vi "InitializeFile.vi"(0 "File Path":path=path "C:/Users/lbignell/Desktop/1 Ton Tank Experiment/Control Software/HDF5/Dummy2.h5", 1 "Thermocouple Location":string[](array[string])=["In Dark Box", "In Room"], 2 "Multiplicity Requirement":u8 max=8, 3 "Run Number":i32, 4 "VME Configuration":T1={"Module Description"=["Bridge", "TDC", "Scaler", "Hodoscope QDC ", "Other QDC", "Digitizer 1", "Digitizer 2", ""], "Module Model"=["V2718", "V775", "V830", "V965A", "V965A", "V1729A", "1729A", ""], "Module Address"=[0, 4026597376, 4026662912, 4026728448, 4026793984, 4026859520, 4026925056]} {"Module Address" format="%.0x"}, 5 "Trigger Bit Descriptions":string[](array[string])=["TrigA", "TrigB", "TrigC", "TrigD"], 6 "LED Frequency (Hz)":dbl, 7 "error in":errorcluster, 8 "Scaler Info":T3={"Chanel Description"=["H0", "H1", "H2", "H3", "H4", "H5", "TrigA", "TrigB", "TrigC", "TrigD", "Ch0", "Ch1", "Ch2", "Ch3", "Ch4", "Ch5", "Ch6", "Ch7"], "Only Hodo?"=[TRUE, TRUE, TRUE, TRUE, TRUE, TRUE, TRUE, TRUE, FALSE, FALSE, FALSE, FALSE, FALSE, FALSE, FALSE, FALSE, FALSE, FALSE]}, 9 "Optional Comments":string, 12 "HV Status":bool, 13 "Material in Tank":string(combo), 14 "Run Type":string(combo), 15 "TDC Info":T3={"Chanel Description"=["H0", "H1", "H2", "H3", "H4", "H5", "TrigA", "TrigB", "TrigC", "TrigD"], "Only Hodo?"=[TRUE, TRUE, TRUE, TRUE, TRUE, TRUE, TRUE, TRUE, FALSE, FALSE]}, 16 "QDC Info":T3={"Chanel Description"=["H0", "H1", "H2", "H3", "H4", "H5"], "Only Hodo?"=[TRUE, TRUE, TRUE, TRUE, TRUE, TRUE]}, 17 "Digitizer Info":T3={"Chanel Description"=["Ch0", "Ch1", "Ch2", "Ch3", "Ch4", "Ch5", "Ch6", "Ch7"], "Only Hodo?"=[FALSE, FALSE, FALSE, FALSE, FALSE, FALSE, FALSE, FALSE]}) -> (20 "File Handle":T2=16777216 format="%.0x", 27 "error out":errorcluster)   [LabVIEW 2014]
uses:
  <vilib>/addons/h5labview2/base/hid_t.ctl
  <vilib>/addons/h5labview2/file/H5Fmode.ctl
  <vilib>/addons/h5labview2/base/lib_path.vi
  <vilib>/addons/h5labview2/base/H5Equery.vi
  DatasetNames.vi
  <vilib>/addons/h5labview2/dataset/H5Dwrite.llb/H5Dwrite.xnode
  <vilib>/addons/h5labview2/file/H5F.lvlib
  <vilib>/addons/h5labview2/group/H5G.lvlib
  <vilib>/addons/h5labview2/props/H5P.lvlib
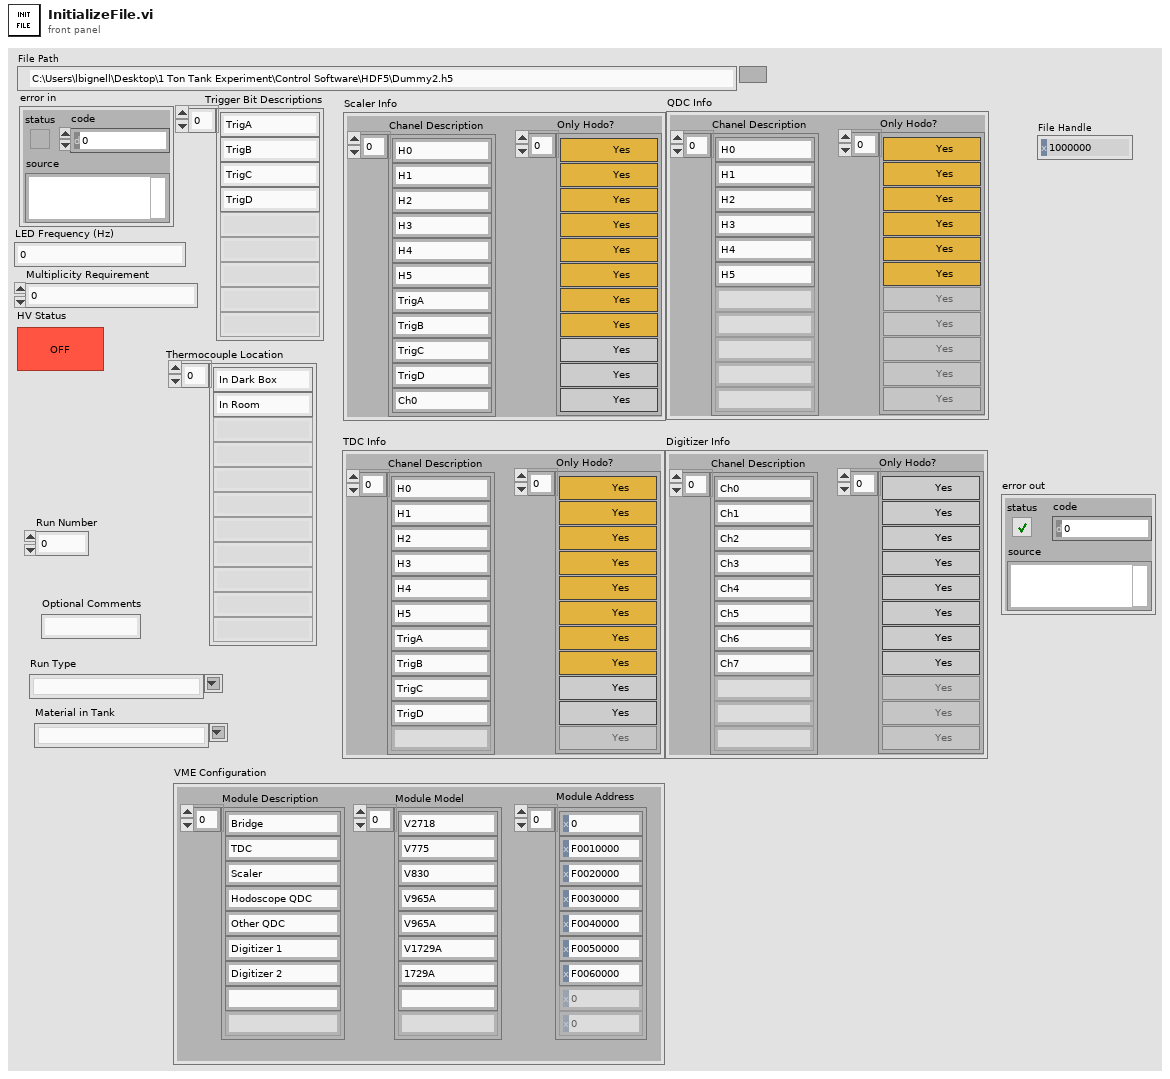
[diagram p1: front panel]
types:
  T1 = cluster{"Module Description":string[], "Module Model":string[], "Module Address":u32[]}
  T2 = typedef "hid_t.ctl" = i32
  T3 = cluster{"Chanel Description":string[], "Only Hodo?":bool[]}
  T4 = typedef "H5F.lvlib/H5Fmode.ctl" = enum16{"read-only", "read-write", "overwrite", "create new", "open or create"}
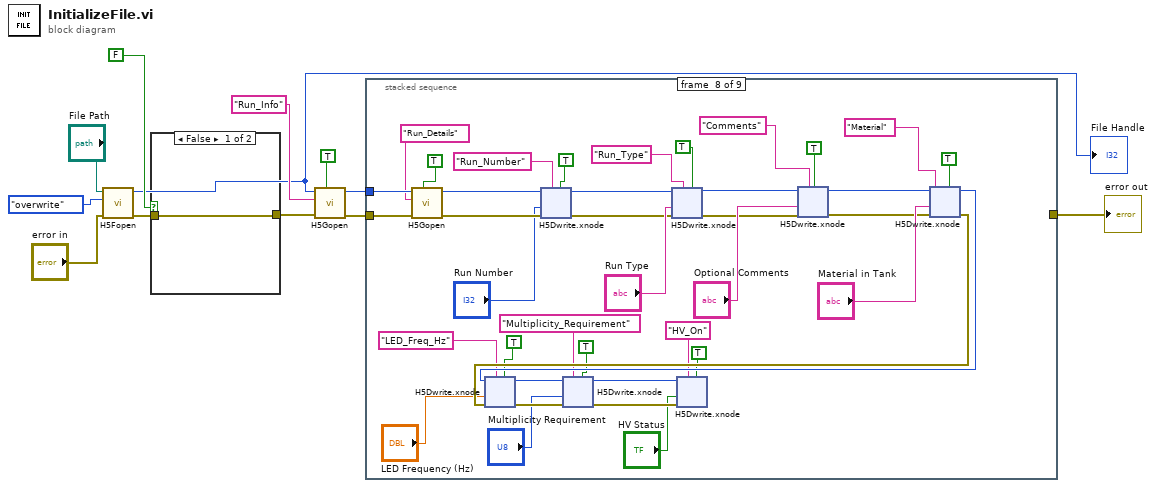
[diagram p0: block diagram]
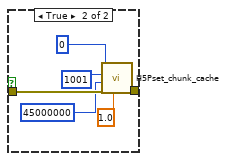
[diagram p2: hidden frame]
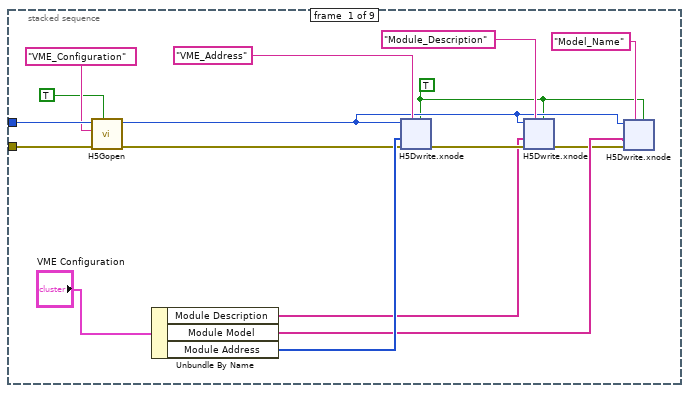
[diagram p3: hidden frame]
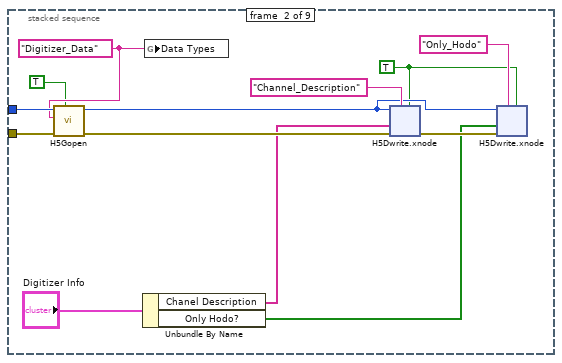
[diagram p4: hidden frame]
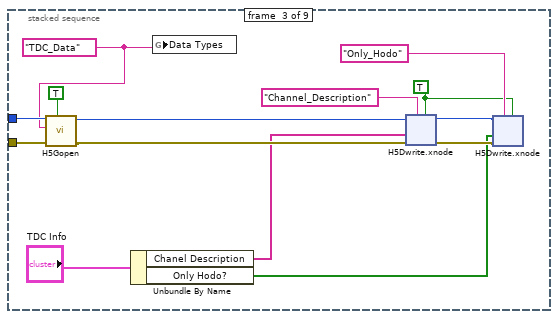
[diagram p5: hidden frame]
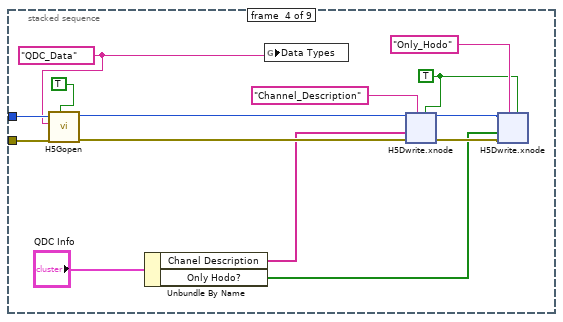
[diagram p6: hidden frame]
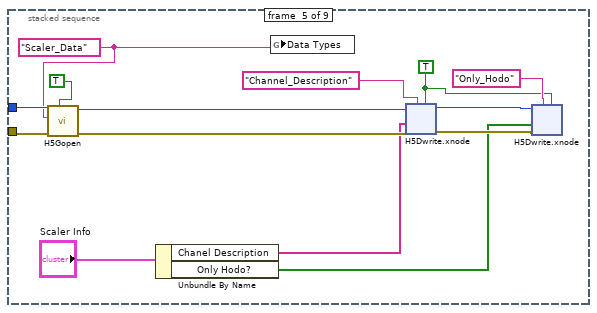
[diagram p7: hidden frame]
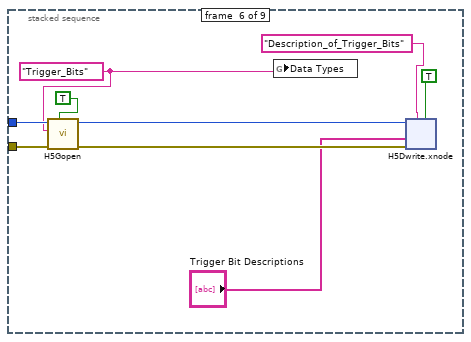
[diagram p8: hidden frame]
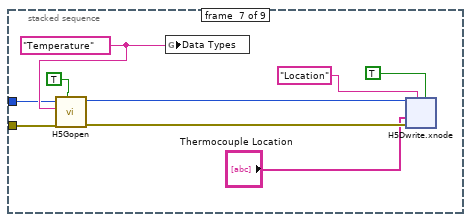
[diagram p9: hidden frame]
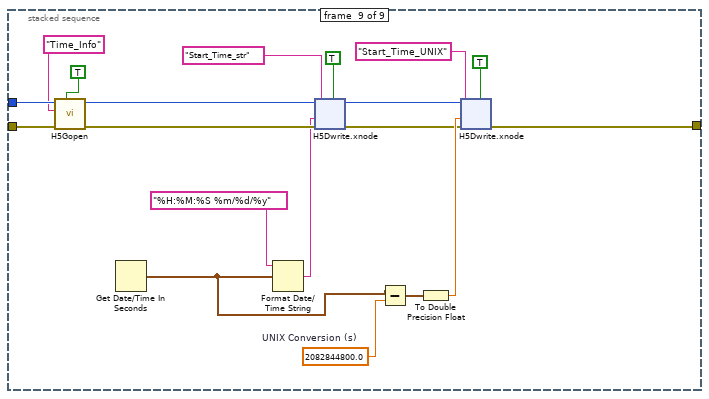
[diagram p10: hidden frame]
diagram:
  n1 = call <vilib>:"H5Fopen.vi"("error in (no error)"="error in", "mode (read-only)"=H5Fmode."overwrite", "path"="File Path") -> ("error out"=w4:errorcluster, "ref out"=w1:T2)  [unwired: 7 in]
  "File Handle" <- w1
  n2 = case shown="False" FALSE {
    tunnel: w4 -> [w13 w19]
    tunnel: [w13 w18] -> w3
    frame False {
    }
    frame True {
      n3 = call <vilib>:"H5Pset_chunk_cache.vi"("w0"=1.0, "error in (no error)"=w19, "nbytes"=u32 45000000, "nslots"=u32 1001, "prop in"=T2 0) -> ("error out"=w18:errorcluster)  [unwired: 5 in, 1 out]
    }
  }
  n4 = call <vilib>:"H5Gopen.vi"("create? (F)"=TRUE, "error in (no error)"=w3, "name"="Run_Info", "ref in"=w1) -> ("error out"=w7:errorcluster, "group out"=w8:T2)  [unwired: 6 in]
  n5 = stacked-sequence {
    tunnel: w8 -> [w31 w100 w149 w200 w250 w296 w317 w380 w525]
    tunnel: w7 -> [w32 w101 w151 w201 w251 w295 w323 w381 w526]
    tunnel: [_ _ _ _ _ _ _ _ w508] -> w6
    frame #0 {
      w21 = TRUE ("replace? (F)")
      n6 = call <vilib>:"H5Gopen.vi"("create? (F)"=TRUE, "error in (no error)"=w32, "name"="VME_Configuration" ("attrib name"), "ref in"=w31) -> ("error out"=w29:errorcluster, "group out"=w25:T2)  [unwired: 6 in]
      n7 = Unbundle By Name("VME Configuration") -> ("Module Description"=w26:string[], "Module Model"=w23:string[], "Module Address"=w33:u32[])
      n8 = xnode "H5Dwrite.xnode"("replace? (F)"=w21, "dataset name"="VME_Address" ("attrib name"), "error in (no error)"=w29, "data"=w33, "ref in"=w25) -> ("error out"=w27:errorcluster)  [unwired: 2 in, 2 out]
      n9 = xnode "H5Dwrite.xnode"("replace? (F)"=w21, "dataset name"="Module_Description" ("attrib name"), "error in (no error)"=w27, "data"=w26, "ref in"=w25) -> ("error out"=w22:errorcluster)  [unwired: 2 in, 2 out]
      n10 = xnode "H5Dwrite.xnode"("replace? (F)"=w21, "dataset name"="Model_Name" ("attrib name"), "error in (no error)"=w22, "data"=w23, "ref in"=w25) -> ()  [unwired: 2 in, 3 out]
    }
    frame #1 {
      w98 = "Digitizer_Data" ("Combo Box")
      w92 = TRUE ("replace? (F)")
      n11 = call <vilib>:"H5Gopen.vi"("create? (F)"=TRUE, "error in (no error)"=w101, "name"=w98, "ref in"=w100) -> ("error out"=w99:errorcluster, "group out"=w94:T2)  [unwired: 6 in]
      n12 = Unbundle By Name("Digitizer Info") -> ("Chanel Description"=w96:string[], "Only Hodo?"=w91:bool[])
      n13 = global write "DatasetNames.vi" "Data Types"(w98) -> ()
      n14 = xnode "H5Dwrite.xnode"("replace? (F)"=w92, "dataset name"="Channel_Description" ("attrib name"), "error in (no error)"=w99, "data"=w96, "ref in"=w94) -> ("error out"=w95:errorcluster)  [unwired: 2 in, 2 out]
      n15 = xnode "H5Dwrite.xnode"("replace? (F)"=w92, "dataset name"="Only_Hodo" ("attrib name"), "error in (no error)"=w95, "data"=w91, "ref in"=w94) -> ()  [unwired: 2 in, 3 out]
    }
    frame #2 {
      w140 = TRUE ("replace? (F)")
      w148 = "TDC_Data" ("Combo Box")
      n16 = call <vilib>:"H5Gopen.vi"("create? (F)"=TRUE, "error in (no error)"=w151, "name"=w148, "ref in"=w149) -> ("error out"=w150:errorcluster, "group out"=w145:T2)  [unwired: 6 in]
      n17 = Unbundle By Name("TDC Info") -> ("Chanel Description"=w144:string[], "Only Hodo?"=w139:bool[])
      n18 = global write "DatasetNames.vi" "Data Types"(w148) -> ()
      n19 = xnode "H5Dwrite.xnode"("replace? (F)"=w140, "dataset name"="Channel_Description" ("attrib name"), "error in (no error)"=w150, "data"=w144, "ref in"=w145) -> ("error out"=w143:errorcluster, "ref out"=w142:i32)  [unwired: 2 in, 1 out]
      n20 = xnode "H5Dwrite.xnode"("replace? (F)"=w140, "dataset name"="Only_Hodo" ("attrib name"), "error in (no error)"=w143, "data"=w139, "ref in"=w142) -> ()  [unwired: 2 in, 3 out]
    }
    frame #3 {
      w190 = TRUE ("replace? (F)")
      w197 = "QDC_Data" ("Combo Box")
      n21 = call <vilib>:"H5Gopen.vi"("create? (F)"=TRUE ("replace? (F)"), "error in (no error)"=w201, "name"=w197, "ref in"=w200) -> ("error out"=w198:errorcluster, "group out"=w199:T2)  [unwired: 6 in]
      n22 = Unbundle By Name("QDC Info") -> ("Chanel Description"=w194:string[], "Only Hodo?"=w189:bool[])
      n23 = global write "DatasetNames.vi" "Data Types"(w197) -> ()
      n24 = xnode "H5Dwrite.xnode"("replace? (F)"=w190, "dataset name"="Channel_Description" ("attrib name"), "error in (no error)"=w198, "data"=w194, "ref in"=w199) -> ("error out"=w193:errorcluster, "ref out"=w192:i32)  [unwired: 2 in, 1 out]
      n25 = xnode "H5Dwrite.xnode"("replace? (F)"=w190, "dataset name"="Only_Hodo" ("attrib name"), "error in (no error)"=w193, "data"=w189, "ref in"=w192) -> ()  [unwired: 2 in, 3 out]
    }
    frame #4 {
      w239 = TRUE ("replace? (F)")
      w247 = "Scaler_Data" ("Combo Box")
      n26 = call <vilib>:"H5Gopen.vi"("create? (F)"=TRUE, "error in (no error)"=w251, "name"=w247, "ref in"=w250) -> ("error out"=w248:errorcluster, "group out"=w249:T2)  [unwired: 6 in]
      n27 = Unbundle By Name("Scaler Info") -> ("Chanel Description"=w244:string[], "Only Hodo?"=w240:bool[])
      n28 = global write "DatasetNames.vi" "Data Types"(w247) -> ()
      n29 = xnode "H5Dwrite.xnode"("replace? (F)"=w239, "dataset name"="Channel_Description" ("attrib name"), "error in (no error)"=w248, "data"=w244, "ref in"=w249) -> ("error out"=w243:errorcluster, "ref out"=w242:i32)  [unwired: 2 in, 1 out]
      n30 = xnode "H5Dwrite.xnode"("replace? (F)"=w239, "dataset name"="Only_Hodo" ("attrib name"), "error in (no error)"=w243, "data"=w240, "ref in"=w242) -> ()  [unwired: 2 in, 3 out]
    }
    frame #5 {
      w292 = "Trigger_Bits" ("Combo Box")
      n31 = call <vilib>:"H5Gopen.vi"("create? (F)"=TRUE ("replace? (F)"), "error in (no error)"=w295, "name"=w292, "ref in"=w296) -> ("error out"=w294:errorcluster, "group out"=w293:T2)  [unwired: 6 in]
      n32 = global write "DatasetNames.vi" "Data Types"(w292) -> ()
      n33 = xnode "H5Dwrite.xnode"("replace? (F)"=TRUE, "dataset name"="Description_of_Trigger_Bits" ("attrib name"), "error in (no error)"=w294, "data"="Trigger Bit Descriptions", "ref in"=w293) -> ()  [unwired: 2 in, 3 out]
    }
    frame #6 {
      w321 = "Temperature" ("Combo Box")
      n34 = call <vilib>:"H5Gopen.vi"("create? (F)"=TRUE ("replace? (F)"), "error in (no error)"=w323, "name"=w321, "ref in"=w317) -> ("error out"=w322:errorcluster, "group out"=w316:T2)  [unwired: 6 in]
      n35 = global write "DatasetNames.vi" "Data Types"(w321) -> ()
      n36 = xnode "H5Dwrite.xnode"("replace? (F)"=TRUE, "dataset name"="Location" ("attrib name"), "error in (no error)"=w322, "data"="Thermocouple Location", "ref in"=w316) -> ()  [unwired: 2 in, 3 out]
    }
    frame #7 {
      n37 = call <vilib>:"H5Gopen.vi"("create? (F)"=TRUE, "error in (no error)"=w381, "name"="Run_Details", "ref in"=w380) -> ("error out"=w361:errorcluster, "group out"=w363:T2)  [unwired: 6 in]
      n38 = xnode "H5Dwrite.xnode"("replace? (F)"=TRUE, "dataset name"="Run_Number", "error in (no error)"=w361, "data"="Run Number", "ref in"=w363) -> ("error out"=w362:errorcluster, "ref out"=w364:i32)  [unwired: 2 in, 1 out]
      n39 = xnode "H5Dwrite.xnode"("replace? (F)"=TRUE, "dataset name"="Run_Type", "error in (no error)"=w362, "data"="Run Type", "ref in"=w364) -> ("error out"=w373:errorcluster, "ref out"=w372:i32)  [unwired: 2 in, 1 out]
      n40 = xnode "H5Dwrite.xnode"("replace? (F)"=TRUE, "dataset name"="Comments", "error in (no error)"=w373, "data"="Optional Comments", "ref in"=w372) -> ("error out"=w368:errorcluster, "ref out"=w369:i32)  [unwired: 2 in, 1 out]
      n41 = xnode "H5Dwrite.xnode"("replace? (F)"=TRUE, "dataset name"="Material", "error in (no error)"=w368, "data"="Material in Tank", "ref in"=w369) -> ("error out"=w356:errorcluster, "ref out"=w357:i32)  [unwired: 2 in, 1 out]
      n42 = xnode "H5Dwrite.xnode"("replace? (F)"=TRUE, "dataset name"="LED_Freq_Hz", "error in (no error)"=w356, "data"="LED Frequency (Hz)", "ref in"=w357) -> ("error out"=w351:errorcluster, "ref out"=w350:i32)  [unwired: 2 in, 1 out]
      n43 = xnode "H5Dwrite.xnode"("replace? (F)"=TRUE, "dataset name"="Multiplicity_Requirement", "error in (no error)"=w351, "data"="Multiplicity Requirement", "ref in"=w350) -> ("error out"=w347:errorcluster, "ref out"=w346:i32)  [unwired: 2 in, 1 out]
      n44 = xnode "H5Dwrite.xnode"("replace? (F)"=TRUE, "dataset name"="HV_On", "error in (no error)"=w347, "data"="HV Status", "ref in"=w346) -> ()  [unwired: 2 in, 3 out]
    }
    frame #8 {
      w517 = 2082844800.0  # UNIX Conversion (s)
      n45 = call <vilib>:"H5Gopen.vi"("create? (F)"=TRUE, "error in (no error)"=w526, "name"="Time_Info", "ref in"=w525) -> ("error out"=w521:errorcluster, "group out"=w522:T2)  [unwired: 6 in]
      n46 = Get Date/Time In Seconds() -> (seconds since 1Jan1904=w516:timestamp)
      n47 = Format Date/Time String(time format string (%c)="%H:%M:%S %m/%d/%y", seconds (now)=w516) -> (date/time string=w518:string)  [unwired: 1 in]
      n48 = xnode "H5Dwrite.xnode"("replace? (F)"=TRUE, "dataset name"="Start_Time_str", "error in (no error)"=w521, "data"=w518, "ref in"=w522) -> ("error out"=w512:errorcluster, "ref out"=w513:i32)  [unwired: 2 in, 1 out]
      n49 = Subtract(x=w516, y=w517) -> (x-y=w515:timestamp)
      n50 = To Double Precision Float(number=w515) -> (double precision float=w514:dbl)
      n51 = xnode "H5Dwrite.xnode"("replace? (F)"=TRUE, "dataset name"="Start_Time_UNIX", "error in (no error)"=w512, "data"=w514, "ref in"=w513) -> ("error out"=w508:errorcluster)  [unwired: 2 in, 2 out]
    }
  }
  "error out" <- w6
